vi "ex02_while_loop.vi"() -> ()   [LabVIEW 2019]
panel:
  out "Numeric 2":i32
  in  "stop 2":bool
  out "Numeric":i32
  in  "stop":bool
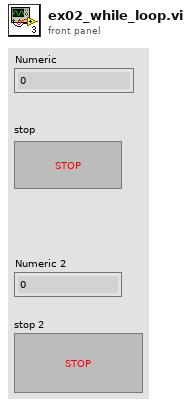
[diagram p1: front panel]
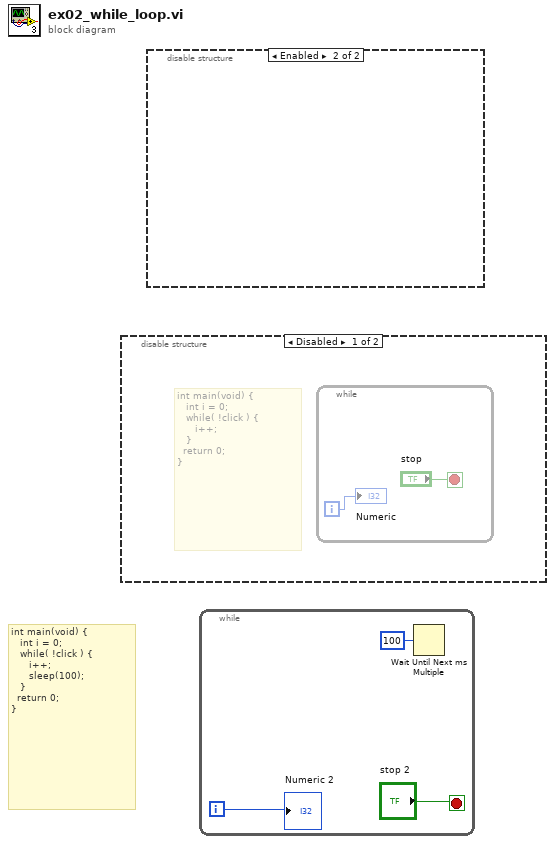
[diagram p0: block diagram]
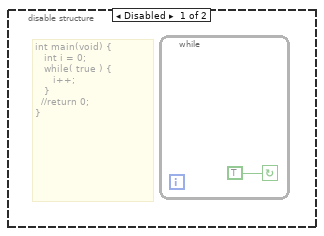
[diagram p3: hidden frame]
diagram:
  # "int main(void) {\n   int i = 0;\n   while( !click ) {\n      i++;\n      sleep(100);\n   }\n  return 0;\n}"
  n1 = disable-structure shown="Disabled" {
    frame Disabled {
      # "int main(void) {\n   int i = 0;\n   while( !click ) {\n      i++;\n   }\n  return 0;\n}"
      n2 = while {
        i -> [w1]
        stop <- "stop" stop-if-true
        "Numeric" <- w1
      }
    }
    frame Enabled {
    }
  }
  n3 = disable-structure shown="Enabled" {
    frame Disabled {
      # "int main(void) {\n   int i = 0;\n   while( true ) {\n      i++;\n   }\n  //return 0;\n}"
      n4 = while {
        stop <- TRUE continue-if-true
      }
    }
    frame Enabled {
    }
  }
  n5 = while {
    i -> [w5]
    stop <- "stop 2" stop-if-true
    n6 = Wait Until Next ms Multiple(millisecond multiple=u32 100) -> ()  [unwired: 1 out]
    "Numeric 2" <- w5
  }
